vi "Get Valid Channels to Update.vi"(8 "error in (no error)":errorcluster, 10 "Data Read":cluster{waveform(dbl)[], string[]}, 11 "Plugin in":refnum<class "StreamReader.lvclass">) -> (0 "error out":errorcluster, 2 "Waveforms Out":waveform(dbl)[](array[waveform]), 3 "Channels Out":string[](array[string]))   [LabVIEW 2024, in "StreamReader.lvlib" / "StreamReader.lvclass"]
uses:
  StreamReader.lvclass
  <vilib>/FlexLogger/SDK/PluginSDK.lvlibp/PEFClasses/SDK/Producer Channel/Producer Channel.lvclass
  <vilib>/FlexLogger/SDK/PluginSDK.lvlibp/PEFClasses/SDK/Plugin/Read Channels.vi
  <vilib>/FlexLogger/SDK/PluginSDK.lvlibp/PEFClasses/SDK/Plugin/Get Valid Producer Channels.vi
  <vilib>/FlexLogger/SDK/PluginSDK.lvlibp/PEFClasses/SDK/Channel/Channel.lvclass
  StreamReader.lvclass/StreamReader.ctl
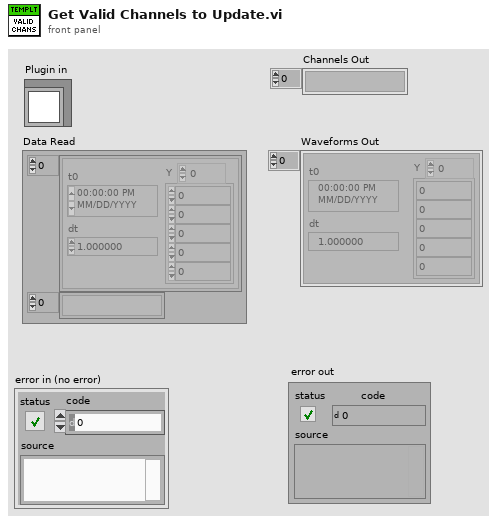
[diagram p1: front panel]
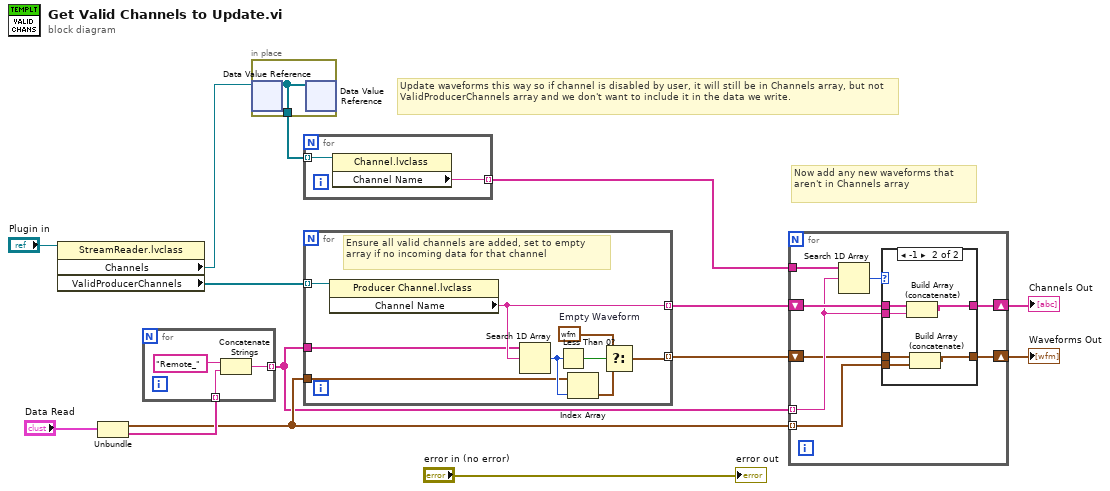
[diagram p0: block diagram]
diagram:
  # "Update waveforms this way so if channel is disabled by user, it will still be in Channels array, but not ValidProducerChannels array and we don't want to include it in the data we write."
  # "Now add any new waveforms that aren't in Channels array"
  n1 = property class="StreamReader.lvclass"(reference="Plugin in") -> ("Channels"=w10:refnum<data-value>, "ValidProducerChannels"=w12:refnum<class "Producer Channel.lvclass">[])  [unwired: 1 in, 2 out]
  n2 = Unbundle("Data Read") -> (w5:waveform(dbl)[], w6:string[])
  n3 = for {
    tunnel: w6 -> [w16] mode=indexing
    tunnel: [w15] -> w3 mode=indexing
    n4 = Concatenate Strings("Remote_" ("string"), w16) -> (w15:string)
  }
  n5 = in-place {
    in-place-border: [w18] -> w9
    n6 = in-place-dvr #1(w10) -> (w18:refnum<class "Channel.lvclass">[])  [unwired: 1 out]
    n7 = in-place-dvr #1(w18) -> ()  [unwired: 2 out]
  }
  n8 = for {
    tunnel: w9 -> [w20] mode=indexing
    tunnel: [w19] -> w8 mode=indexing
    n9 = property class="Channel.lvclass"(reference=w20) -> ("Channel Name"=w19:string)  [unwired: 1 in, 2 out]
  }
  n10 = for {
    tunnel: w12 -> [w29] mode=indexing
    tunnel: [w28] -> w7 mode=indexing
    tunnel: w3 -> [w27]
    tunnel: w5 -> [w23]
    tunnel: [w21] -> w4 mode=indexing
    w25 = waveform(dbl) {"t0"=timestamp(0 s since 1904-01-01), "dt"=1.0, "Y"=[]}  # Empty Waveform
    # "Ensure all valid channels are added, set to empty array if no incoming data for that channel"
    n11 = property class="Producer Channel.lvclass"(reference=w29) -> ("Channel Name"=w28:string)  [unwired: 1 in, 2 out]
    n12 = Search 1D Array(1D array=w27, element=w28) -> (index of element=w24:i32)  [unwired: 1 in]
    n13 = Less Than 0?(x=w24) -> (x < 0?=w26:bool)
    n14 = Index Array(array=w23, index=w24) -> (element=w22:waveform(dbl))
    n15 = Select(t=w25, s=w26, f=w22) -> (s? t:f=w21:waveform(dbl))
  }
  n16 = for {
    tunnel: w5 -> [w30] mode=indexing
    tunnel: w3 -> [w34] mode=indexing
    tunnel: w8 -> [w37]
    shift-right: [w33] -> w2
    shift-left: w7 -> [w35]
    shift-right: [w31] -> w1
    shift-left: w4 -> [w32]
    n17 = Search 1D Array(1D array=w37, element=w34) -> (index of element=w36:i32)  [unwired: 1 in]
    n18 = case shown="-1" w36 {
      tunnel: w35 -> [w39 w45]
      tunnel: w34 -> [_ w44]
      tunnel: [w39 w43] -> w33
      tunnel: w32 -> [w38 w42]
      tunnel: [w38 w40] -> w31
      tunnel: w30 -> [_ w41]
      frame 0, Default {
      }
      frame -1 {
        n19 = Build Array (concatenate)(w45, w44) -> (w43:string[])
        n20 = Build Array (concatenate)(w42, w41) -> (w40:waveform(dbl)[])
      }
    }
  }
  "Channels Out" <- w2
  "Waveforms Out" <- w1
  "error out" <- "error in (no error)"
